vi "Corr Transducers Save INFO.vi"(8 "error in":errorcluster, 10 "transducer info":T1, 11 "Path":path) -> (0 "error out":errorcluster)   [LabVIEW 2020]
doc: "Transducer correction INFO saver."
uses:
  Corr Transducer INFO Record.ctl
  Corr Transducer INFO Item.ctl
  Corr CSV Template.ctl
  <vilib>/Utility/error.llb/Error Cluster From Error Code.vi
  octave/infolib/String.vi
  octave/infolib/EXT.vi
  <vilib>/ErrorRing/Error Ring.xnode
  octave/infolib/infolib.lvlib
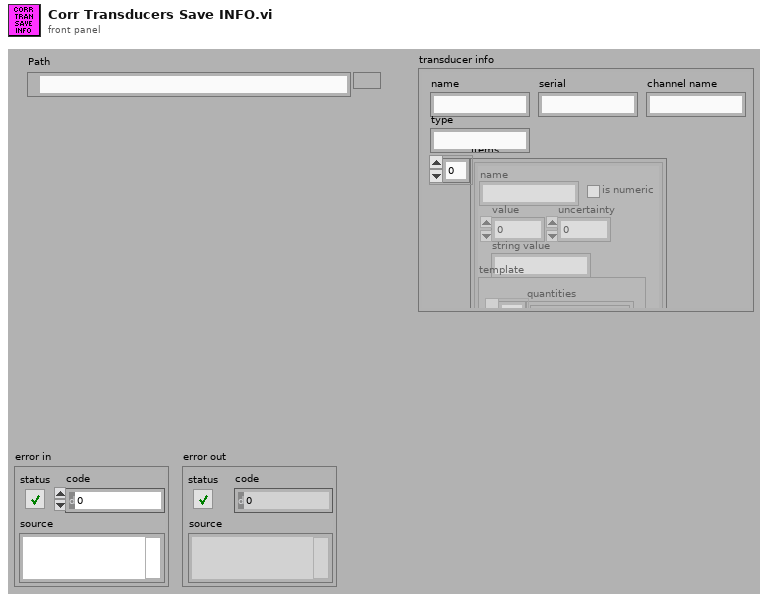
[diagram p1: front panel]
types:
  T1 = typedef "Corr Transducer INFO Record.ctl" = cluster{"name":string, "serial":string, "channel name":string, "items":T2[], "type":string}
  T2 = typedef "Corr Transducer INFO Item.ctl" = cluster{"name":string, "is numeric":bool, "value":dbl, "uncertainty":dbl, "string value":string, "template":T3, "info":string}
  T3 = typedef "Corr CSV Template.ctl" = cluster{"quantities":string[], "y-axis":string, "x-axis":string}
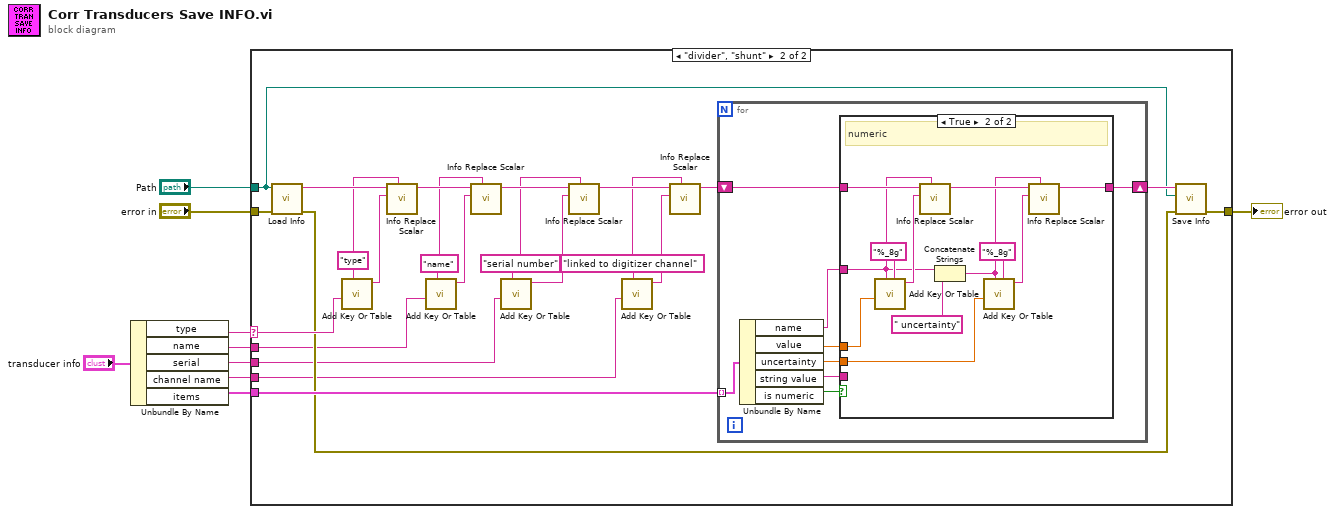
[diagram p0: block diagram]
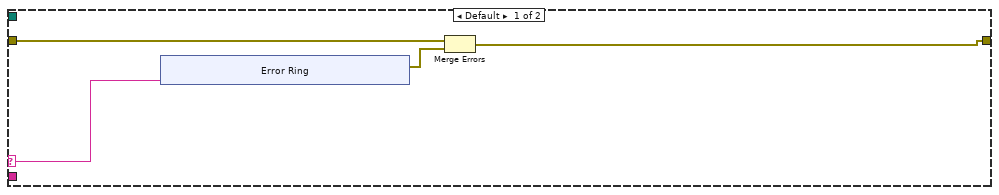
[diagram p2: hidden frame]
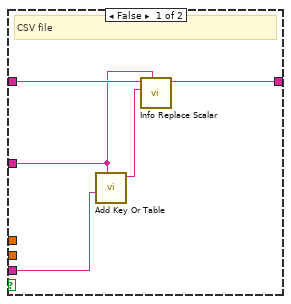
[diagram p3: hidden frame]
diagram:
  n1 = Unbundle By Name("transducer info") -> ("type"=w8:string, "name"=w7:string, "serial"=w6:string, "channel name"=w5:string, "items"=w2:T2[])
  n2 = case shown="\"divider\", \"shunt\"" w8 {
    selector: w8 -> [w13 w43]
    tunnel: w7 -> [_ w23]
    tunnel: w6 -> [_ w22]
    tunnel: w5 -> [_ w21]
    tunnel: "Path" -> [_ w25]
    tunnel: "error in" -> [w12 w37]
    tunnel: w2 -> [_ w31]
    tunnel: [w10 w24] -> w1
    frame Default {
      n3 = xnode "Error Ring"("parameter 0"=w13) -> ("error out"=w11:errorcluster)
      n4 = Merge Errors(w12, w11) -> (w10:errorcluster)
    }
    frame "divider", "shunt" {
      w33 = "linked to digitizer channel" ("key description")
      w35 = "serial number" ("key description")
      w40 = "type" ("key description")
      w38 = "name" ("key description")
      n5 = call "Load Info.vi"("error in"=w37, "filename"=w25) -> ("error out"=w26:errorcluster, "info data"=w42:string)  [unwired: 8 in]
      n6 = call-poly "Add Key Or Table.vi"("key description"=w40, "string"=w43) -> ("info data out"=w41:string)  [unwired: 8 in, 1 out]
      n7 = call "Info Replace Scalar.vi"("key description to replace"=w40, "info data to paste"=w41, "info data in"=w42) -> ("info data out"=w39:string)  [unwired: 8 in]
      n8 = call-poly "Add Key Or Table.vi"("key description"=w38, "string"=w23) -> ("info data out"=w30:string)  [unwired: 8 in, 1 out]
      n9 = call "Info Replace Scalar.vi"("key description to replace"=w38, "info data to paste"=w30, "info data in"=w39) -> ("info data out"=w36:string)  [unwired: 8 in]
      n10 = call-poly "Add Key Or Table.vi"("key description"=w35, "string"=w22) -> ("info data out"=w29:string)  [unwired: 8 in, 1 out]
      n11 = call "Info Replace Scalar.vi"("key description to replace"=w35, "info data to paste"=w29, "info data in"=w36) -> ("info data out"=w34:string)  [unwired: 8 in]
      n12 = call-poly "Add Key Or Table.vi"("key description"=w33, "string"=w21) -> ("info data out"=w28:string)  [unwired: 8 in, 1 out]
      n13 = call "Info Replace Scalar.vi"("key description to replace"=w33, "info data to paste"=w28, "info data in"=w34) -> ("info data out"=w32:string)  [unwired: 8 in]
      n14 = for {
        shift-right: [w45] -> w27
        shift-left: w32 -> [w49]
        tunnel: w31 -> [w51] mode=indexing
        n15 = Unbundle By Name(w51) -> ("name"=w48:string, "value"=w47:dbl, "uncertainty"=w46:dbl, "string value"=w44:string, "is numeric"=w50:bool)
        n16 = case shown="True" w50 {
          tunnel: w49 -> [w55 w68]
          tunnel: w48 -> [w52 w61]
          tunnel: w47 -> [_ w67]
          tunnel: w46 -> [_ w59]
          tunnel: [w54 w57] -> w45
          tunnel: w44 -> [w53 _]
          frame False {
            # "CSV file"
            n17 = call-poly "Add Key Or Table.vi"("key description"=w52, "string"=w53) -> ("info data out"=w56:string)  [unwired: 8 in, 1 out]
            n18 = call "Info Replace Scalar.vi"("key description to replace"=w52, "info data to paste"=w56, "info data in"=w55) -> ("info data out"=w54:string)  [unwired: 8 in]
          }
          frame True {
            # "numeric"
            n19 = call-poly "Add Key Or Table.vi"("format string (%.;%#_20f)"="%_8g" ("format string (%_20f)"), "key description"=w61, "numeric"=w67) -> ("info data out"=w66:string)  [unwired: 7 in, 1 out]
            n20 = call "Info Replace Scalar.vi"("key description to replace"=w61, "info data to paste"=w66, "info data in"=w68) -> ("info data out"=w62:string)  [unwired: 8 in]
            n21 = Concatenate Strings(w61, " uncertainty" ("string")) -> (w58:string)
            n22 = call-poly "Add Key Or Table.vi"("format string (%.;%#_20f)"="%_8g" ("format string (%_20f)"), "key description"=w58, "numeric"=w59) -> ("info data out"=w63:string)  [unwired: 7 in, 1 out]
            n23 = call "Info Replace Scalar.vi"("key description to replace"=w58, "info data to paste"=w63, "info data in"=w62) -> ("info data out"=w57:string)  [unwired: 8 in]
          }
        }
      }
      n24 = call "Save Info.vi"("error in"=w26, "filename"=w25, "info data"=w27) -> ("error out"=w24:errorcluster)  [unwired: 8 in]
    }
  }
  "error out" <- w1
